vi "ProtoBuff - Read How Many Bytes Available to Read.vi"(8 "error in (no error)":errorcluster, 11 "TCP Network Connection in":refnum<k5>) -> (0 "error out":errorcluster, 2 "Bytes Available":u32, 3 "TCP Network Connection out":refnum<k5>)   [LabVIEW 2020]
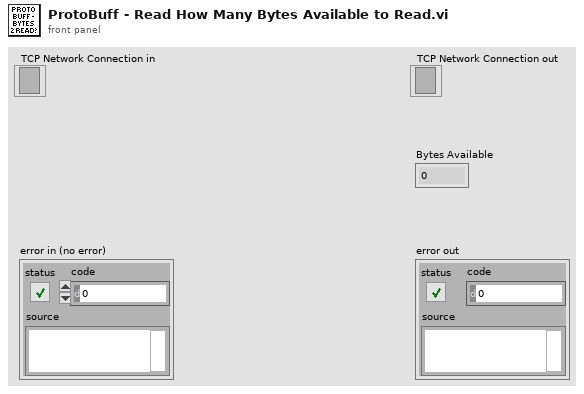
[diagram p1: front panel]
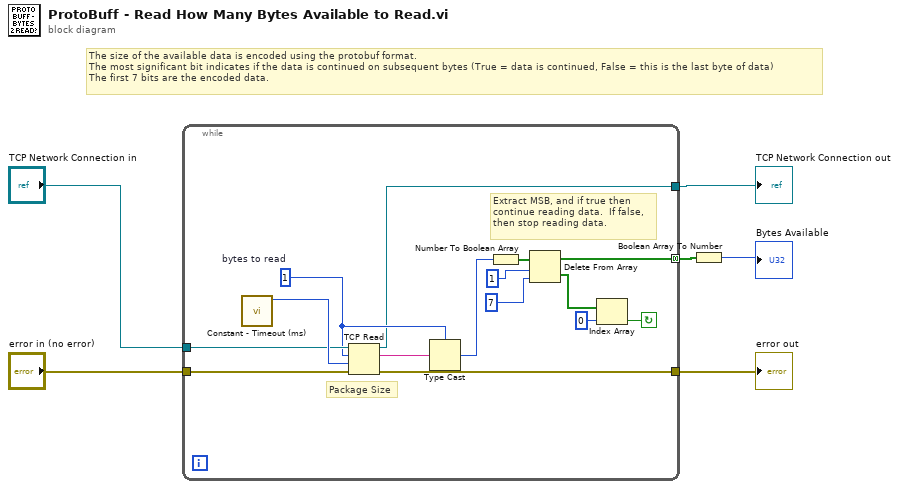
[diagram p0: block diagram]
diagram:
  # "The size of the available data is encoded using the protobuf format.  \nThe most significant bit indicates if the data is continued on subsequent bytes (True = data is continued, False = this is the last byte of data)\nThe first 7 bits are the encoded data."
  n1 = while {
    tunnel: "TCP Network Connection in" -> [w19]
    tunnel: [w10] -> w6
    tunnel: [w9] -> w4
    tunnel: [w8] -> w3 mode=concatenating
    tunnel: "error in (no error)" -> [w7]
    stop <- w11 continue-if-true
    w18 = u8 1  # bytes to read
    # "Extract MSB, and if true then\ncontinue reading data.  If false,\nthen stop reading data."
    # "Package Size"
    n2 = call "Constant - Timeout (ms).vi"() -> ("timeout (ms)"=w20:i32)  [unwired: 11 in]
    n3 = TCP Read(connection ID=w19, bytes to read=w18, error in (no error)=w7, 9:w20) -> (connection ID out=w10:refnum<k5>, data out=w21:string, error out=w9:errorcluster)  [unwired: 1 in]
    n4 = Type Cast(type=w18, x=w21) -> (*(type *) &x=w17:u8)
    n5 = Number To Boolean Array(number=w17) -> (Boolean array=w16:bool[])
    n6 = Delete From Array(array=w16, length=1, index=7) -> (deleted portion=w13:bool[], array with subset deleted=w8:bool[])
    n7 = Index Array(array=w13, index=0) -> (element=w11:bool)
  }
  "TCP Network Connection out" <- w6
  "error out" <- w4
  n8 = Boolean Array To Number(Boolean array=w3) -> (number=→"Bytes Available":u32)
